vi "Port for Service.vi"(8 "error in (no error)":errorcluster, 9 "type":T1, 10 "services":T2[](array[typedef])) -> (0 "error out":errorcluster, 2 "port":i32)   [LabVIEW 2020, in "Vecto.lvlib"]
uses:
  Vecto.lvlib
  lv-volatus/messages/Service/Data.ctl
  lv-volatus/messages/ServiceType/Enumeration.ctl
  lv-volatus/messages/ServiceType/ServiceType.lvlib
  lv-volatus/messages/Service/Service.lvlib
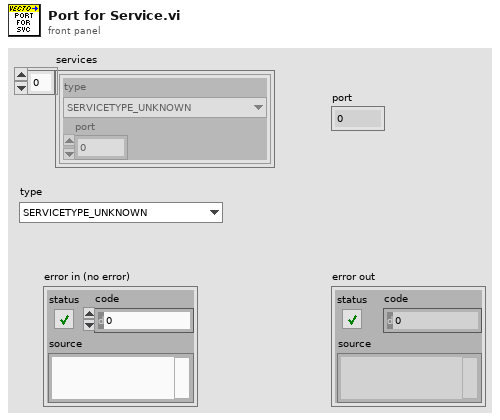
[diagram p1: front panel]
types:
  T1 = typedef "ServiceType.lvlib/Enumeration.ctl" = enum16{"SERVICETYPE_UNKNOWN", "SERVICETYPE_TCPSERVER", "SERVICETYPE_HTTPSERVER"}
  T2 = typedef "Service.lvlib/Data.ctl" = cluster{"type":T1, "port":i32}
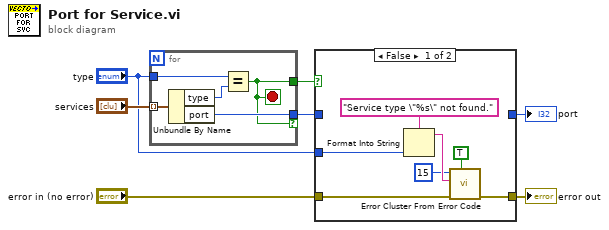
[diagram p0: block diagram]
diagram:
  n1 = for {
    tunnel: "services" -> [w12] mode=indexing
    tunnel: "type" -> [w10]
    tunnel: [w9] -> w6 if=w8
    tunnel: [w8] -> w5
    stop <- w8 stop-if-true
    n2 = Unbundle By Name(w12) -> ("type"=w11:T1, "port"=w9:i32)
    n3 = Equal?(x=w10, y=w11) -> (x = y?=w8:bool)
  }
  n4 = case shown="False" w5 {
    tunnel: w6 -> [_ w21]
    tunnel: [_ w21] -> w4
    tunnel: "error in (no error)" -> [w17 w20]
    tunnel: "type" -> [w19 _]
    tunnel: [w13 w20] -> w1
    frame False {
      n5 = Format Into String(format string="Service type \"%s\" not found.", w19) -> (resulting string=w16:string)  [unwired: 2 in, 1 out]
      n6 = call <vilib>:"Error Cluster From Error Code.vi"("show call chain? (False)"=TRUE, "error in (no error)"=w17, "error message (\"\")"=w16, "error code (0)"=15) -> ("error out"=w13:errorcluster)  [unwired: 5 in]
    }
    frame True {
    }
  }
  "error out" <- w1
  "port" <- w4
